vi "CreateRenderer.vi"(8 "No Error":errorcluster, 10 "Name (\"\": NULL)":string, 11 "Window [SDL_Window *]":T1 format="%.0x") -> (0 "Error Out":errorcluster, 3 "Renderer [SDL_Renderer *]":T2 format="%.0x")   [LabVIEW 2026, in "SDL3.lvlib" / "Render.lvlib"]
doc: "<B>Summary</B>\nCreate a 2D rendering context for a window.\n\n<B>Remarks</B>\nIf you want a specific renderer, you can specify its name here. A list of available renderers can be obtained by calling SDL_GetRenderDriver multiple times, with indices from 0 to SDL_GetNumRenderDrivers()-1. If you don't need a specific renderer, specify NULL and SDL will attempt to choose the best option for you, based on what is available on the user's system.\n\nBy default the rendering size matches the window size in pixels, but you can call SDL_SetRenderLogicalPresentation() to change the content size and scaling options."
uses:
  Render.lvlib
  <vilib>/Utility/error.llb/Error Cluster From Error Code.vi
  Error/Error.lvlib
  Lib/SDL3.dll
  SDL_Renderer--pointer.ctl
  Video/SDL_Window--pointer.ctl
  Video/Video.lvlib
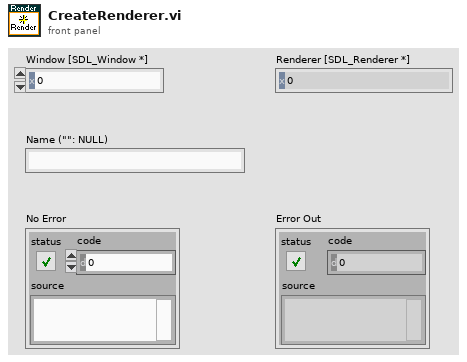
[diagram p1: front panel]
types:
  T1 = typedef "SDL3.lvlib/Video.lvlib/SDL_Window--pointer.ctl" = i64
  T2 = typedef "SDL3.lvlib/Render.lvlib/SDL_Renderer--pointer.ctl" = i64
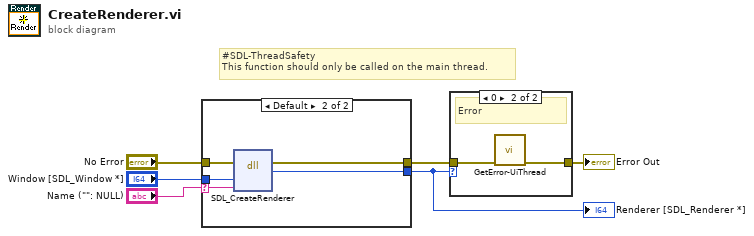
[diagram p0: block diagram]
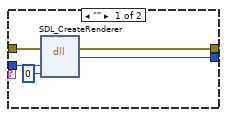
[diagram p2: hidden frame]
diagram:
  # "#SDL-ThreadSafety\nThis function should only be called on the main thread."
  n1 = case shown="Default" "Name (\"\": NULL)" {
    selector: "Name (\"\": NULL)" -> [_ w14]
    tunnel: "No Error" -> [w11 w16]
    tunnel: [w10 w15] -> w1
    tunnel: [w9 w13] -> w3
    tunnel: "Window [SDL_Window *]" -> [w8 w12]
    frame "" {
      n2 = dll-call lib="C:/Users/saukko/Dev/LV-SDL3/Sources/SDL3/Lib/SDL3.*" fn="SDL_CreateRenderer"(error in=w11, "window"=w8, "title"=i64 0) -> (error out=w10:errorcluster, "return type"=w9:i64)  [unwired: 4 in, 1 out]
    }
    frame Default {
      n3 = dll-call lib="C:/Users/saukko/Dev/LV-SDL3/Sources/SDL3/Lib/SDL3.*" fn="SDL_CreateRenderer"(error in=w16, "window"=w12, "title"=w14) -> (error out=w15:errorcluster, "return type"=w13:i64)  [unwired: 4 in, 1 out]
    }
  }
  "Renderer [SDL_Renderer *]" <- w3
  n4 = case shown="0" w3 {
    tunnel: w1 -> [w17 w19]
    tunnel: [w17 w18] -> w5
    frame Default {
      # "Ok"
    }
    frame 0 {
      # "Error"
      n5 = call "GetError-UiThread.vi"("No Error"=w19) -> ("error out"=w18:errorcluster)  [unwired: 10 in]
    }
  }
  "Error Out" <- w5
